vi "FPGA Read IRQ Context Queue.vi"(8 "error in (no error)":errorcluster, 11 "FPGA Interface Base in":refnum<class "FPGA Interface Base.lvclass">) -> (0 "error out":errorcluster, 2 "IRQ Context Queue":refnum<queue>, 3 "FPGA Interface Base out":refnum<class "FPGA Interface Base.lvclass">)   [LabVIEW 2010, in "FPGA Interface Base.lvclass"]
uses:
  <userlib>/_FPGA Interface Advanced Tools/FPGA Interface Base/FPGA Interface Base.lvclass
  <userlib>/_FPGA Interface Advanced Tools/FPGA Interface Base/FPGA Interface Base.lvclass/FPGA Interface Base.ctl
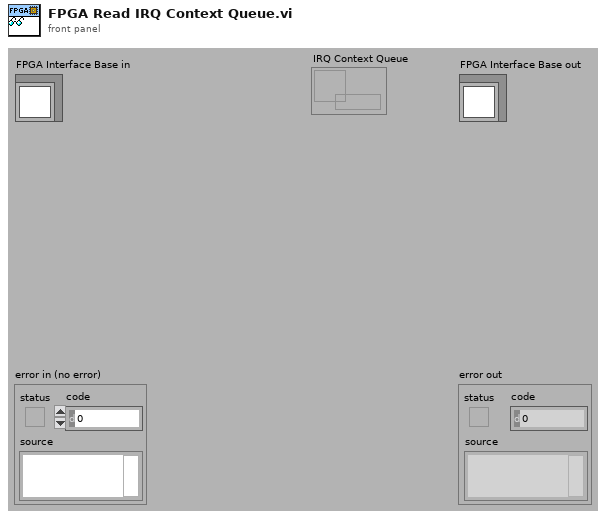
[diagram p1: front panel]
types:
  T1 = typedef "FPGA Interface Base.lvclass/FPGA Session.ctl" = refnum<data-value>
  T2 = typedef "FPGA Interface Base.lvclass/FPGA Session Data.ctl" = cluster{"Session Out":u32, "Indicator Scalars":T3, "Indicator Arrays":T5, "Control Scalars":T3, "Control Arrays":T5, "TargetToHost FIFO Channels":T7, "HostToTarget FIFO Channels":T7, "All FIFOs":T8[], "IRQ Context Queue":refnum<queue>}
  T3 = typedef "FPGA Bitfile Utility.lvlib/Scalar Register Set.ctl" = cluster{"Boolean":T4[], "I8":T4[], "I16":T4[], "I32":T4[], "I64":T4[], "U8":T4[], "U16":T4[], "U32":T4[], "U64":T4[]}
  T4 = typedef "FPGA Bitfile Utility.lvlib/Scalar Register.ctl" = cluster{"Address":u32, "Name":string}
  T5 = typedef "FPGA Bitfile Utility.lvlib/Array Register Set.ctl" = cluster{"Boolean":T6[], "I8":T6[], "I16":T6[], "I32":T6[], "I64":T6[], "U8":T6[], "U16":T6[], "U32":T6[], "U64":T6[]}
  T6 = typedef "FPGA Bitfile Utility.lvlib/Array Register.ctl" = cluster{"Address":u32, "Num Elements":u32, "Name":string}
  T7 = typedef "FPGA Bitfile Utility.lvlib/FIFO Channel Set.ctl" = cluster{"Boolean":T8[], "I8":T8[], "I16":T8[], "I32":T8[], "I64":T8[], "U8":T8[], "U16":T8[], "U32":T8[], "U64":T8[]}
  T8 = typedef "FPGA Bitfile Utility.lvlib/FIFO Channel.ctl" = cluster{"Physical Channel":u32, "Name":string}
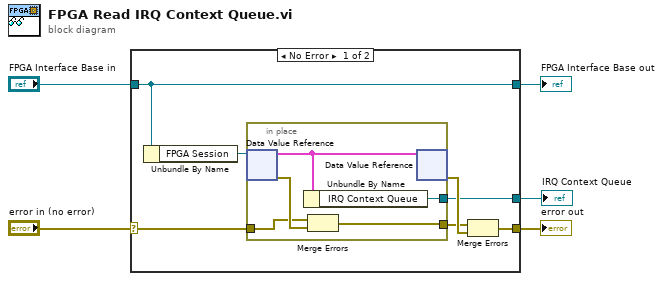
[diagram p0: block diagram]
diagram:
  n1 = case shown="No Error" "error in (no error)" {
    selector: "error in (no error)" -> [w6 w18]
    tunnel: [w7 w18] -> w4
    tunnel: [w12 w19] -> w2
    tunnel: "FPGA Interface Base in" -> [w12 w19]
    tunnel: [w8 _] -> w1
    frame No Error {
      n2 = Unbundle By Name(w12) -> ("FPGA Session"=w9:T1)
      n3 = in-place {
        in-place-border: w6 -> [w16]
        in-place-border: [w14] -> w8
        in-place-border: [w13] -> w10
        n4 = in-place-dvr #1(w9) -> (w15:T2, w17:errorcluster)
        n5 = Unbundle By Name(w15) -> ("IRQ Context Queue"=w14:refnum<queue>)
        n6 = Merge Errors(w16, w17) -> (w13:errorcluster)
        n7 = in-place-dvr #1(w15) -> (w11:errorcluster)  [unwired: 1 out]
      }
      n8 = Merge Errors(w10, w11) -> (w7:errorcluster)
    }
    frame Error {
    }
  }
  "error out" <- w4
  "FPGA Interface Base out" <- w2
  "IRQ Context Queue" <- w1
